vi "ASDAcquire.vi"(0 "TCP Network Connection Refnum":refnum<k5>, 5 "Acquire":bool, 11 "error in (no error)":errorcluster) -> (4 "Header Code":i32, 6 "Error Code":i32, 10 "Spectrum Data":sgl[](array[numeric]), 15 "error out":errorcluster)   [LabVIEW 2010]
panel:
  # "This is a Sub-VI of ASDTCPDemo.vi"
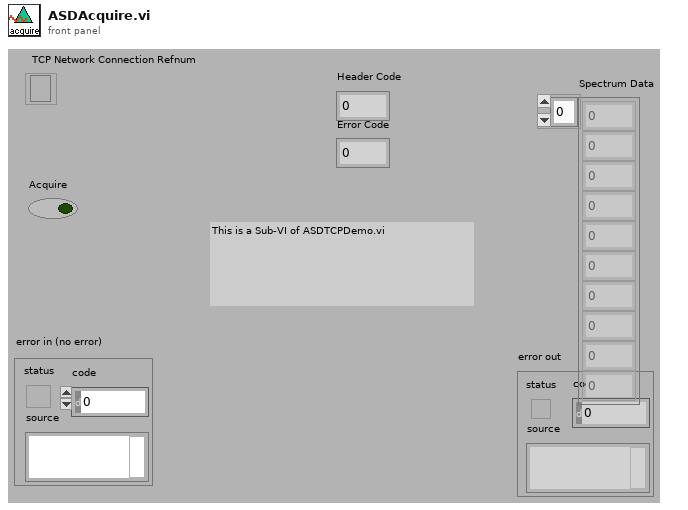
[diagram p1: front panel]
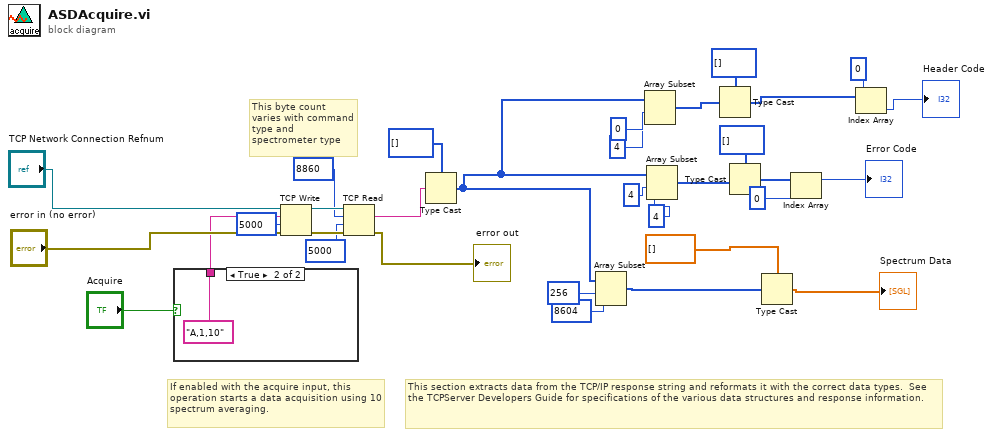
[diagram p0: block diagram]
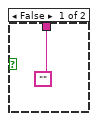
[diagram p2: hidden frame]
diagram:
  # "This byte count varies with command type and spectrometer type"
  # "This section extracts data from the TCP/IP response string and reformats it with the correct data types.  See the TCPServer Developers Guide for specifications of the various data structures and response information."
  # "If enabled with the acquire input, this operation starts a data acquisition using 10 spectrum averaging."
  n1 = case shown="True" "Acquire" {
    tunnel: ["" "A,1,10"] -> w25
    frame False {
    }
    frame True {
    }
  }
  n2 = TCP Write(connection ID="TCP Network Connection Refnum", data in=w25, error in (no error)="error in (no error)", 9:5000 ("timeout ms (25000)")) -> (connection ID out=w28:refnum<k5>, error out=w29:errorcluster)  [unwired: 1 out]
  n3 = TCP Read(connection ID=w28, bytes to read=8860, error in (no error)=w29, 9:5000 ("timeout ms (25000)")) -> (data out=w27:string, error out=→"error out":errorcluster)  [unwired: 1 in, 1 out]
  n4 = Type Cast(type=u8[] [], x=w27) -> (*(type *) &x=w5:u8[])
  n5 = Array Subset(array=w5, index=256, length=8604) -> (w24:u8[])
  n6 = Array Subset(array=w5, index=0 ("start index (0)"), length=4) -> (w12:u8[])
  n7 = Array Subset(array=w5, index=4, length=4 ("index")) -> (w8:u8[])
  n8 = Type Cast(type=i32[] [], x=w12) -> (*(type *) &x=w11:i32[])
  n9 = Type Cast(type=i32[] [], x=w8) -> (*(type *) &x=w9:i32[])
  n10 = Type Cast(type=sgl[] [], x=w24) -> (*(type *) &x=→"Spectrum Data":sgl[])
  n11 = Index Array(array=w9, index=0) -> (element=→"Error Code":i32)
  n12 = Index Array(array=w11, index=0) -> (element=→"Header Code":i32)
